vi "Lab07.vi"() -> ()   [LabVIEW 2024]
panel:
  in  "DampFactor":dbl(slide) scale=0.0..10.0
  in  "Proportional":bool
  in  "SetPoint":dbl(slide) scale=15.0..35.0 scale format="%#_2g"
  in  "COMM_Name":refnum<visa-resource-name>
  in  "stop":bool
  out "Warm":bool
  out "Cold":bool
  out "Waveform Chart":dbl(graph)
  out "Thermometer, C":dbl(slide) scale=0.0..100.0
  out "R, KOhms":dbl format="%1.2f"
  out "AtoD, Hex":i32 format="%04x"
  out "SCC, V":dbl format="%01.3f"
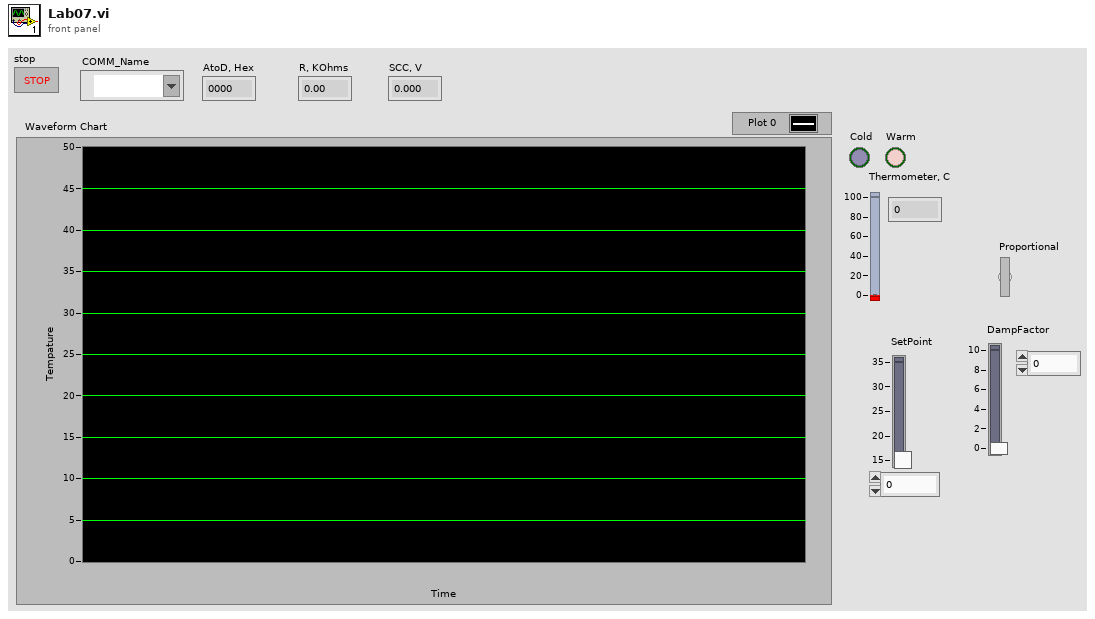
[diagram p1: front panel]
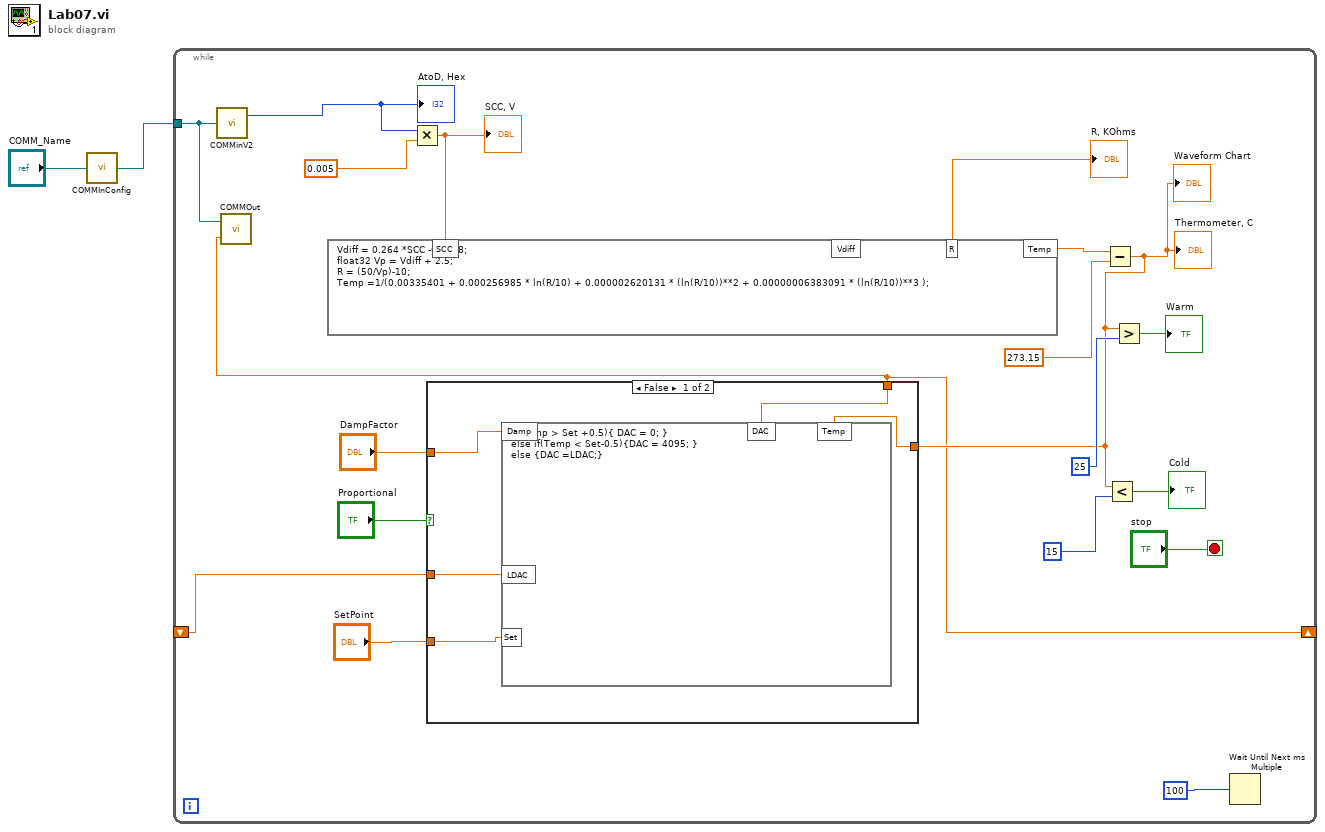
[diagram p0: block diagram]
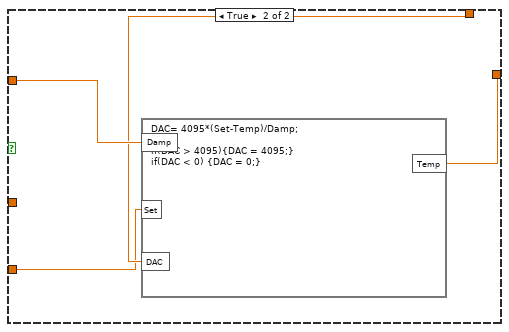
[diagram p2: hidden frame]
diagram:
  n1 = call "COMMInConfig.vi"("COMM_in"="COMM_Name") -> ("COMM_Name"=w1:refnum<visa-resource-name>)
  n2 = while {
    tunnel: w1 -> [w8]
    shift-right: [w3] -> _
    shift-left: _ -> [w4]
    stop <- "stop" stop-if-true
    n3 = call "COMMinV2.vi"("VISA resource name"=w8) -> ("AtoDOut"=w11:i16)  [unwired: 1 out]
    "AtoD, Hex" <- w11
    n4 = Multiply(x=w11, y=0.005) -> (x*y=w21:dbl)
    "SCC, V" <- w21
    n5 = formula code="Vdiff = 0.264 *SCC -0.8268;\nfloat32 Vp = Vdiff + 2.5;\nR = (50/Vp)-10;\nTemp =1/(0.00335401 + 0.000256985 * ln(R/10) + 0.000002620131 * (ln(R/10))**2 + 0.00000006383091 * (ln(R/10))**3 );"("SCC"=w21) -> ("R"=→"R, KOhms":dbl, "Temp"=w7:dbl)  [unwired: 1 out]
    n6 = Subtract(x=w7, y=273.15) -> (x-y=w5:dbl)
    "Thermometer, C" <- w5
    "Waveform Chart" <- w5
    n7 = case shown="False" "Proportional" {
      tunnel: w5 -> [w25 w29]
      tunnel: "DampFactor" -> [w26 w30]
      tunnel: [w23 w28] -> w3
      tunnel: "SetPoint" -> [w24 w27]
      tunnel: w4 -> [w22 _]
      frame False {
        n8 = formula code="if(Temp > Set +0.5){ DAC = 0; }\nelse if(Temp < Set-0.5){DAC = 4095; }\nelse {DAC =LDAC;}"("Temp"=w25, "Set"=w24, "Damp"=w26, "LDAC"=w22) -> ("DAC"=w23:dbl)
      }
      frame True {
        n9 = formula code="DAC= 4095*(Set-Temp)/Damp;\n\nif(DAC > 4095){DAC = 4095;}\nif(DAC < 0) {DAC = 0;}"("Damp"=w30, "Temp"=w29, "Set"=w27) -> ("DAC"=w28:dbl)
      }
    }
    n10 = call "COMMOut.vi"("Numeric"=w3, "VISA resource name"=w8) -> ()
    n11 = Less?(x=w5, y=15) -> (x < y?=→"Cold":bool)
    n12 = Greater?(x=w5, y=25) -> (0:→"Warm":bool)
    n13 = Wait Until Next ms Multiple(millisecond multiple=100) -> ()  [unwired: 1 out]
  }
